vi "fpga_next_target.vi"(0 "scanning":bool, 1 "scan config":T3, 3 "abort":bool, 5 "measure completed?":bool, 7 "move completed?":bool, 9 "inrange?":bool, 11 "scan (manual)":bool, 12 "Read Target":bool=TRUE, 13 "initial positions (manual)":T2, 14 "index (manual)":T1) -> (4 "target":T2, 6 "index":T1, 10 "scanning":bool, 15 "new target":bool)   [LabVIEW 2021]
doc: "Calculate the next target.\n\nThe next target will be calculated from the initial scan condition and current index. When the scan is turned off, the vi try to get new scanning initial parameters. During the scan, target will be updated only after the measurement was completed at the previous cycle, or forced backward scan. \n\nPlease also see the documentation of \"fpga_get_scan_ini.vi\"."
uses:
  fpga_dtype_sgl_8ch.ctl
  fpga_dtype_scan_config.ctl
  fpga_dtype_index.ctl
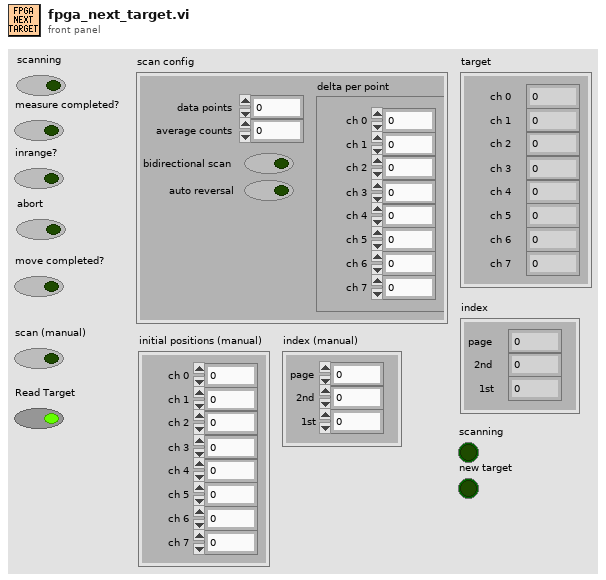
[diagram p1: front panel]
types:
  T1 = typedef "fpga_dtype_index.ctl" = cluster{"page":i16, "2nd":i16, "1st":i16}
  T2 = typedef "fpga_dtype_sgl_8ch.ctl" = cluster{"ch 0":sgl, "ch 1":sgl, "ch 2":sgl, "ch 3":sgl, "ch 4":sgl, "ch 5":sgl, "ch 6":sgl, "ch 7":sgl}
  T3 = typedef "fpga_dtype_scan_config.ctl" = cluster{"data points":i16, "average counts":i16, "delta per point":T2, "bidirectional scan":bool, "auto reversal":bool}
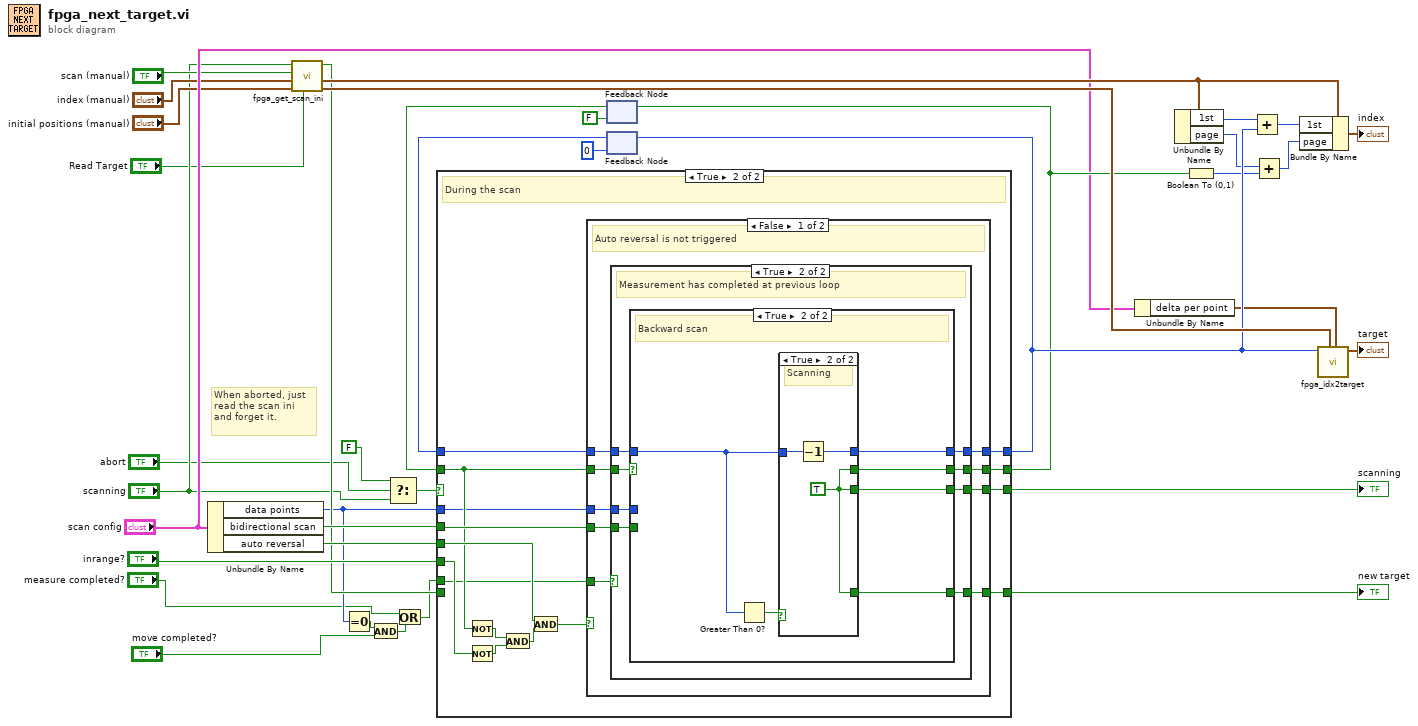
[diagram p0: block diagram]
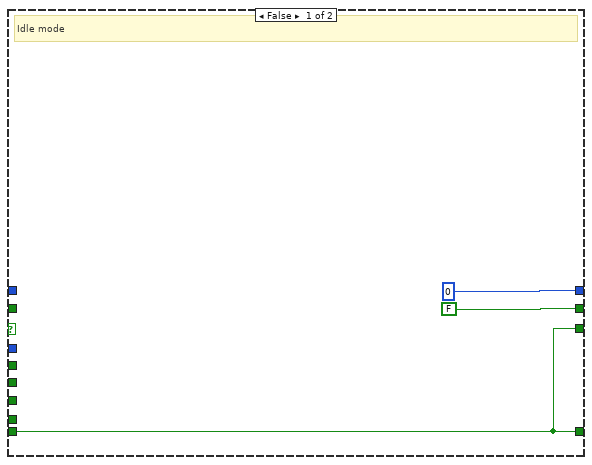
[diagram p2: hidden frame]
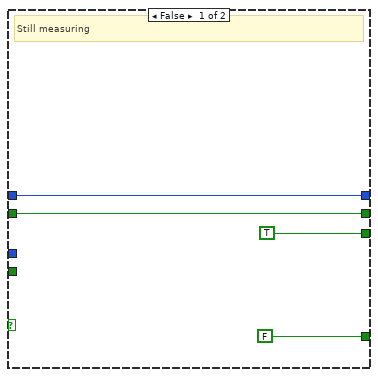
[diagram p3: hidden frame]
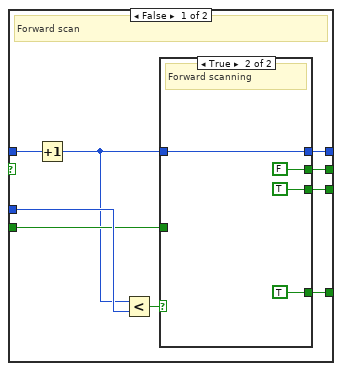
[diagram p4: hidden frame]
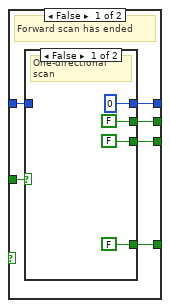
[diagram p5: hidden frame]
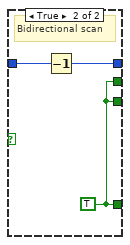
[diagram p6: hidden frame]
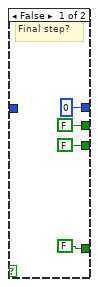
[diagram p7: hidden frame]
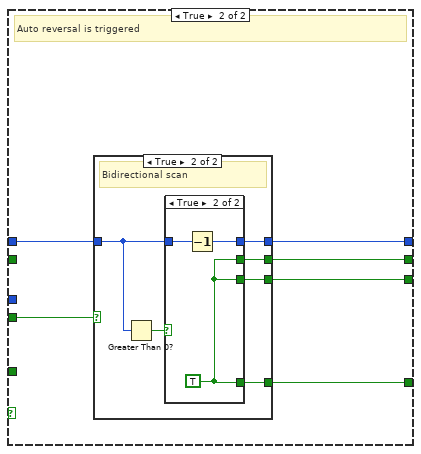
[diagram p8: hidden frame]
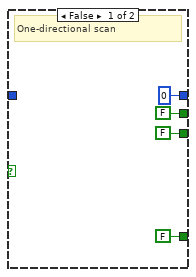
[diagram p9: hidden frame]
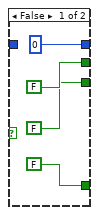
[diagram p10: hidden frame]
diagram:
  # "When aborted, just read the scan ini and forget it."
  n1 = Unbundle By Name("scan config") -> ("data points"=w11:i16, "bidirectional scan"=w18:bool, "auto reversal"=w17:bool)
  n2 = call "fpga_get_scan_ini.vi"("Read Target"="Read Target", "initial positions (manual)"="initial positions (manual)", "index offset (manual)"="index (manual)", "scan (manual)"="scan (manual)", "scanning"="scanning") -> ("initial positions"=w34:T2, "index offfset"=w31:T1, "new scan?"=w15:bool)  [unwired: 4 in]
  n3 = Equal To 0?(x=w11) -> (x = 0?=w4:bool)
  n4 = And(x=w4, y="move completed?") -> (x .and. y?=w2:bool)
  n5 = Select(t=FALSE, s="abort", f="scanning") -> (s? t:f=w8:bool)
  n6 = Or(x="measure completed?", y=w2) -> (x .or. y?=w9:bool)
  n7 = feedback #1(FALSE) -> (w20:bool)
  n8 = feedback #2(i16 0) -> (w35:i16)
  n9 = case shown="True" w8 {
    tunnel: [w38 w46] -> w26
    tunnel: [w38 w45] -> w27
    tunnel: [i16 0 w44] -> w29
    tunnel: [FALSE w47] -> w22
    tunnel: w20 -> [_ w43]
    tunnel: w11 -> [_ w41]
    tunnel: w18 -> [_ w49]
    tunnel: w17 -> [_ w51]
    tunnel: "inrange?" -> [_ w55]
    tunnel: w9 -> [_ w42]
    tunnel: w35 -> [_ w48]
    tunnel: w15 -> [w38 _]
    frame False {
      # "Idle mode"
    }
    frame True {
      # "During the scan"
      n10 = Not(x=w43) -> (.not. x?=w54:bool)
      n11 = Not(x=w55) -> (.not. x?=w53:bool)
      n12 = And(x=w54, y=w53) -> (x .and. y?=w52:bool)
      n13 = And(x=w51, y=w52) -> (x .and. y?=w50:bool)
      n14 = case shown="False" w50 {
        tunnel: w49 -> [w56 w121]
        tunnel: w48 -> [w63 w120]
        tunnel: [w60 w119] -> w47
        tunnel: [w58 w118] -> w46
        tunnel: [w59 w117] -> w45
        tunnel: [w61 w116] -> w44
        tunnel: w43 -> [w64 _]
        tunnel: w42 -> [w62 _]
        tunnel: w41 -> [w57 _]
        frame False {
          # "Auto reversal is not triggered"
          n15 = case shown="True" w62 {
            tunnel: w64 -> [w67 w76]
            tunnel: w63 -> [w68 w75]
            tunnel: [w68 w74] -> w61
            tunnel: [w67 w73] -> w60
            tunnel: [TRUE w72] -> w59
            tunnel: [FALSE w71] -> w58
            tunnel: w57 -> [_ w70]
            tunnel: w56 -> [_ w69]
            frame False {
              # "Still measuring"
            }
            frame True {
              # "Measurement has completed at previous loop"
              n16 = case shown="True" w76 {
                tunnel: w75 -> [w81 w107]
                tunnel: [w82 w106] -> w74
                tunnel: [w80 w105] -> w73
                tunnel: [w79 w104] -> w72
                tunnel: [w78 w103] -> w71
                tunnel: w70 -> [w85 _]
                tunnel: w69 -> [w83 _]
                frame False {
                  # "Forward scan"
                  n17 = Increment(x=w81) -> (x+1=w77:i16)
                  n18 = Less?(x=w77, y=w85) -> (x < y?=w84:bool)
                  n19 = case shown="True" w84 {
                    tunnel: w83 -> [w91 _]
                    tunnel: [w90 w99] -> w82
                    tunnel: w77 -> [w89 w99]
                    tunnel: [w88 FALSE] -> w80
                    tunnel: [w87 TRUE] -> w79
                    tunnel: [w86 TRUE] -> w78
                    frame False {
                      # "Forward scan has ended"
                      n20 = case shown="False" w91 {
                        tunnel: [i16 0 w96] -> w90
                        tunnel: w89 -> [_ w98]
                        tunnel: [FALSE w97] -> w88
                        tunnel: [FALSE w97] -> w87
                        tunnel: [FALSE w97] -> w86
                        frame False {
                          # "One-directional scan"
                        }
                        frame True {
                          w97 = TRUE
                          # "Bidirectional scan"
                          n21 = Decrement(x=w98) -> (x-1=w96:i16)
                        }
                      }
                    }
                    frame True {
                      # "Forward scanning"
                    }
                  }
                }
                frame True {
                  # "Backward scan"
                  n22 = Greater Than 0?(x=w107) -> (x > 0?=w108:bool)
                  n23 = case shown="True" w108 {
                    tunnel: w107 -> [_ w115]
                    tunnel: [i16 0 w114] -> w106
                    tunnel: [FALSE w113] -> w105
                    tunnel: [FALSE w113] -> w104
                    tunnel: [FALSE w113] -> w103
                    frame False {
                      # "Final step?"
                    }
                    frame True {
                      w113 = TRUE
                      # "Scanning"
                      n24 = Decrement(x=w115) -> (x-1=w114:i16)
                    }
                  }
                }
              }
            }
          }
        }
        frame True {
          # "Auto reversal is triggered"
          n25 = case shown="True" w121 {
            tunnel: w120 -> [_ w130]
            tunnel: [FALSE w129] -> w119
            tunnel: [FALSE w128] -> w118
            tunnel: [FALSE w127] -> w117
            tunnel: [i16 0 w126] -> w116
            frame False {
              # "One-directional scan"
            }
            frame True {
              # "Bidirectional scan"
              n26 = Greater Than 0?(x=w130) -> (x > 0?=w131:bool)
              n27 = case shown="True" w131 {
                tunnel: w130 -> [_ w138]
                tunnel: [FALSE w137] -> w129
                tunnel: [FALSE w137] -> w128
                tunnel: [FALSE w137] -> w127
                tunnel: [i16 0 w136] -> w126
                frame False {
                }
                frame True {
                  w137 = TRUE
                  n28 = Decrement(x=w138) -> (x-1=w136:i16)
                }
              }
            }
          }
        }
      }
    }
  }
  "scanning" <- w27
  "new target" <- w26
  n29 = feedback-in #1(w22) -> ()
  n30 = feedback-in #2(w29) -> ()
  n31 = Unbundle By Name("scan config") -> ("delta per point"=w28:T2)
  n32 = Unbundle By Name(w31) -> ("1st"=w33:i16, "page"=w24:i16)
  n33 = Boolean To (0,1)(Boolean=w22) -> (0, 1=w25:i16)
  n34 = Add(x=w33, y=w29) -> (x+y=w32:i16)
  n35 = Add(x=w24, y=w25) -> (x+y=w23:i16)
  n36 = Bundle By Name(cluster=w31, "1st"=w32, "page"=w23) -> (→"index":T1)
  n37 = call "fpga_idx2target.vi"("delta"=w28, "initial position"=w34, "idx"=w29) -> ("target"=→"target":T2)  [unwired: 8 in]
